vi "GEOM_CorrectionAddition.vi"(8 "ini shift":u32, 9 "iniX":u32, 10 "sorted amplifiers":T1[](array[typedef]) {"fliped" items=["none", "horizontal", "vertical"]; "type" items=["LL", "LR", "UL", "UR"]}) -> (0 "out shift":u32, 1 "out x":u32, 2 "amplifiers out":T1[](array[typedef]) {"fliped" items=["none", "horizontal", "vertical"]; "type" items=["LL", "LR", "UL", "UR"]})   [LabVIEW 2016]
uses:
  GEOM_Amplifier.ctl
  GEOM_AmpType.ctl
  GEOM_ROI.ctl
  GEOM_Coords.ctl
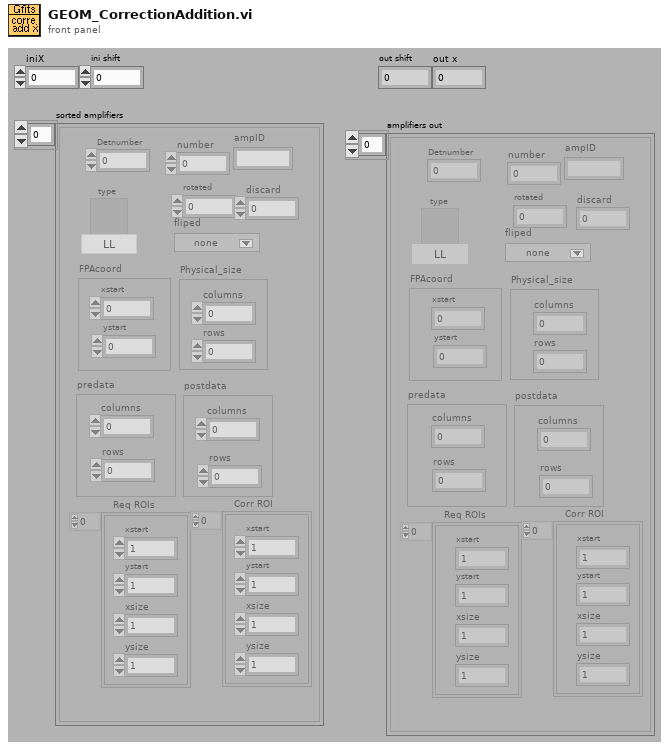
[diagram p1: front panel]
types:
  T1 = typedef "GEOM_Amplifier.ctl" = cluster{"number":i32, "type":T2, "rotated":i16, "fliped":u16, "FPAcoord":cluster{"xstart":i32, "ystart":i32}, "Physical_size":cluster{"columns":i32, "rows":i32}, "predata":cluster{"columns":i32, "rows":i32}, "postdata":cluster{"columns":i32, "rows":i32}, "Req ROIs":T3, "Corr ROI":T3, "Detnumber":i32, "ampID":string, "discard":i32}
  T2 = typedef "GEOM_AmpType.ctl" = u16
  T3 = typedef "GEOM_ROI.ctl" = T4[]
  T4 = typedef "GEOM_Coords.ctl" = cluster{"xstart":u32, "ystart":u32, "xsize":u32, "ysize":u32}
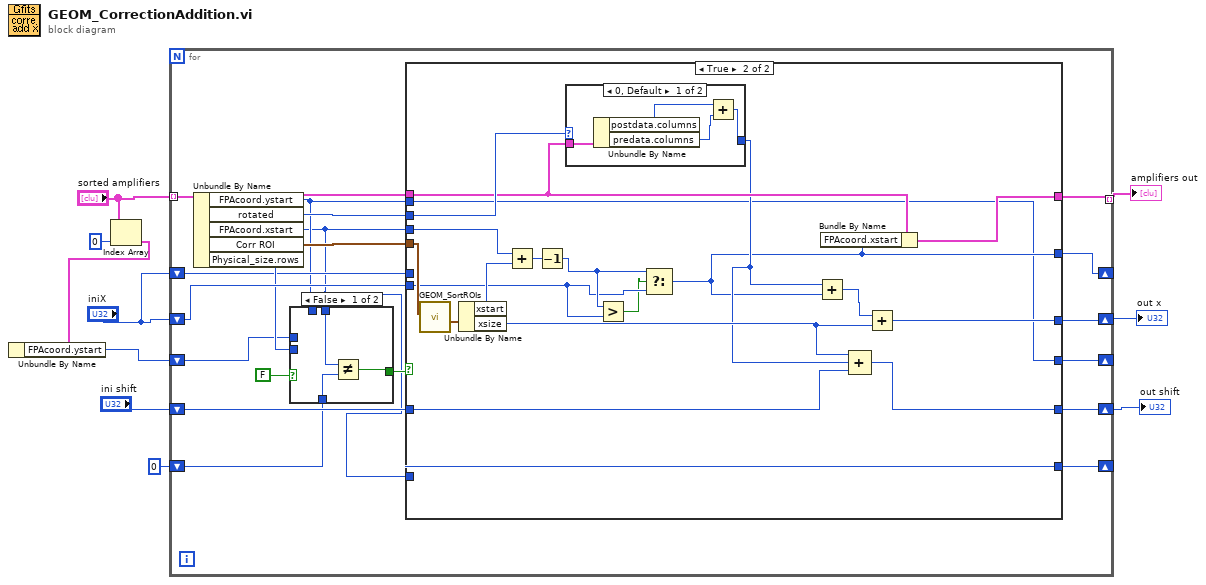
[diagram p0: block diagram]
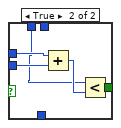
[diagram p2: hidden frame]
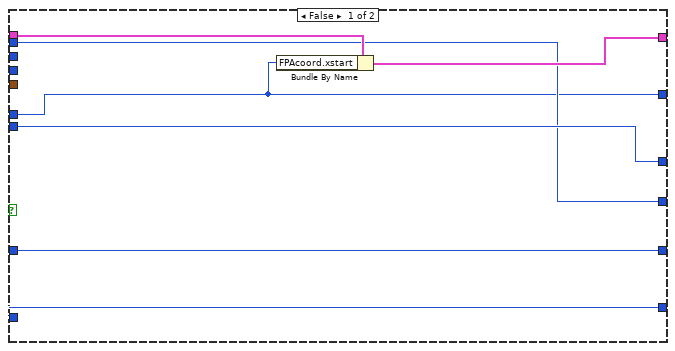
[diagram p3: hidden frame]
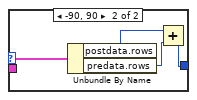
[diagram p4: hidden frame]
diagram:
  n1 = Index Array(array="sorted amplifiers", index=0) -> (element=w3:T1)
  n2 = Unbundle By Name(w3) -> ("FPAcoord.ystart"=w2:i32)
  n3 = for {
    tunnel: "sorted amplifiers" -> [w25] mode=indexing
    shift-right: [w27] -> w7
    shift-left: "iniX" -> [w22]
    tunnel: [w29] -> w10 mode=indexing
    shift-right: [w24] -> w8
    shift-left: "ini shift" -> [w23]
    shift-right: [w20] -> _
    shift-left: 0 ("ystart") -> [w12]
    shift-right: [w21] -> _
    shift-left: "iniX" -> [w17]
    shift-right: [w19] -> _
    shift-left: w2 -> [w15]
    n4 = Unbundle By Name(w25) -> ("FPAcoord.ystart"=w14:i32, "rotated"=w28:i16, "FPAcoord.xstart"=w11:i32, "Corr ROI"=w26:T3, "Physical_size.rows"=w18:i32)
    n5 = case shown="False" FALSE {
      tunnel: w18 -> [_ w37]
      tunnel: [w32 w36] -> w16
      tunnel: w15 -> [_ w34]
      tunnel: w14 -> [_ w33]
      tunnel: w11 -> [w31 _]
      tunnel: w12 -> [w30 _]
      frame False {
        n6 = Not Equal?(x=w31, y=w30) -> (x != y?=w32:bool)
      }
      frame True {
        n7 = Add(x=w34, y=w37) -> (x+y=w35:i32)
        n8 = Less?(x=w33, y=w35) -> (x < y?=w36:bool)
      }
    }
    n9 = case shown="True" w16 {
      tunnel: [w43 w64] -> w29
      tunnel: w28 -> [_ w63]
      tunnel: [w42 w61] -> w27
      tunnel: w26 -> [_ w60]
      tunnel: w25 -> [w44 w56]
      tunnel: [w41 w53] -> w24
      tunnel: w23 -> [w41 w52]
      tunnel: w22 -> [w42 w50]
      tunnel: w11 -> [_ w48]
      tunnel: [w38 w47] -> w21
      tunnel: w11 -> [w40 w46]
      tunnel: [w40 w46] -> w20
      tunnel: w14 -> [w39 w45]
      tunnel: [w39 w45] -> w19
      tunnel: w17 -> [w38 _]
      frame False {
        n10 = Bundle By Name(cluster=w44, "FPAcoord.xstart"=w38) -> (w43:T1)
      }
      frame True {
        n11 = call "GEOM_SortROIs.vi"("ROIs"=w60) -> ("Extreme Coords"=w59:T4)  [unwired: 10 out]
        n12 = Unbundle By Name(w59) -> ("xstart"=w58:u32, "xsize"=w55:u32)
        n13 = Add(x=w48, y=w58) -> (x+y=w57:u32)
        n14 = Decrement(x=w57) -> (x-1=w51:u32)
        n15 = case shown="0, Default" w63 {
          tunnel: w56 -> [w68 w72]
          tunnel: [w65 w69] -> w54
          frame 0, Default {
            n16 = Unbundle By Name(w68) -> ("postdata.columns"=w67:i32, "predata.columns"=w66:i32)
            n17 = Add(x=w67, y=w66) -> (x+y=w65:i32)
          }
          frame -90, 90 {
            n18 = Unbundle By Name(w72) -> ("postdata.rows"=w71:i32, "predata.rows"=w70:i32)
            n19 = Add(x=w71, y=w70) -> (x+y=w69:i32)
          }
        }
        n20 = Greater?(x=w51, y=w50) -> (0:w49:bool)
        n21 = Select(t=w51, s=w49, f=w50) -> (s? t:f=w47:u32)
        n22 = Add(x=w54, y=w47) -> (x+y=w62:u32)
        n23 = Bundle By Name(cluster=w56, "FPAcoord.xstart"=w47) -> (w64:T1)
        n24 = Compound Arithmetic op=ADD(w55, w54, w52) -> (w53:u32)
        n25 = Add(x=w62, y=w55) -> (x+y=w61:u32)
      }
    }
  }
  "amplifiers out" <- w10
  "out shift" <- w8
  "out x" <- w7
